vi "Initialize Attributes.vi"(8 "Error In":errorcluster, 10 "Attribute Data":variant, 11 "KIT-QVA in":refnum<class "KIT-QVA.lvclass">) -> (0 "Error Out":errorcluster, 2 "Found?":bool, 3 "KIT-QVA out":refnum<class "KIT-QVA.lvclass">)   [LabVIEW 2014, in "KIT-QVA.lvlib" / "KIT-QVA.lvclass"]
doc: "Initialize object attribute.\n\nUnique resources should be allocated elsewhere!"
uses:
  KIT-QVA.lvclass
  HardwareStatus-PVEnum.ctl
  RackStatus-PVEnum.ctl
  DetectorStatus-PVEnum.ctl
  CSPP_Core/Classes/CS++ProcessVariables/ProcessVariable/PV.lvclass
  CSPP_Core/Classes/CS++ProcessVariables/ProcessVariable/PV.lvclass/PV.ctl
  CSPP_Core/Actors/CS++BaseActor/CS++BaseActor.lvclass/CS++BaseActor.ctl
  KIT-QVA.lvclass/KIT-QVA.ctl
  CSPP_Core/Classes/CS++ProcessVariables/ProcessVariable/Write PV URL.vi
  CSPP_Core/Classes/CS++ProcessVariables/ProcessVariable/Write Type Descriptor.vi
  CSPP_Core/Classes/CS++ProcessVariables/ProcessVariable/Write Name.vi
  CSPP_Core/Actors/CS++DeviceActor/CS++DeviceActor.lvclass
  CSPP_Core/Classes/CS++BaseClasses/Factory/CS++Factory.lvclass
  CSPP_Core/Libraries/Utilities/CS++Utilities.lvlib
  CSPP_Core/Actors/CS++BaseActor/CS++BaseActor.lvclass
  CSPP_Core/Classes/CS++ProcessVariables/CS++ProcessVariables.lvlib
panel:
  in  "Detector-PVEnum":T1
  in  "Rack-PVEnum":T2
  in  "Hardware-PVEnum":T3
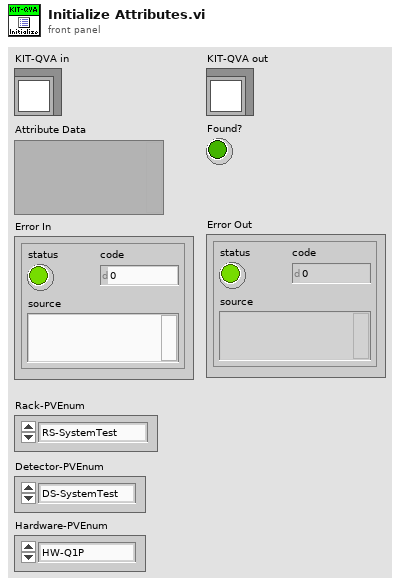
[diagram p1: front panel]
types:
  T1 = typedef "KIT-QVA.lvlib/KIT-QVA.lvclass/DetectorStatus-PVEnum.ctl" = enum16{"DS-SystemTest", "DS-TestMode", "DS-Fault", "DS-Quench", "DS-UTFault", "DS-BusError", "DS-SystemFault", "DS-ADCRaw", "DS-ADCV"}
  T2 = typedef "KIT-QVA.lvlib/KIT-QVA.lvclass/RackStatus-PVEnum.ctl" = enum16{"RS-SystemTest", "RS-TestMode", "RS-Fault", "RS-Quench", "RS-UTFault", "RS-BusError", "RS-SystemFault", "RS-ControlMode", "RS-AveragedT"}
  T3 = typedef "KIT-QVA.lvlib/KIT-QVA.lvclass/HardwareStatus-PVEnum.ctl" = enum16{"HW-Q1P", "HW-Q1M", "HW-Q2P", "HW-Q2M", "HW-Mute", "HW-STestBit", "HW-QD1", "HW-QD2"}
  T4 = cluster{"Q1+":bool, "Q1-":bool, "Q2+":bool, "Q2-":bool, "Mute":bool, "STest-Bit":bool, "QD1":bool, "QD2":bool}
  T5 = cluster{"System Test":bool, "Test Mode":bool, "Fault":bool, "Quench":bool, "U/T Fault":bool, "Bus Error":bool, "System Fault":bool, "Reserved":bool}
  T6 = cluster{"System Test":bool, "Test Mode":bool, "Fault":bool, "Quench":bool, "U/T Fault":bool, "Bus Error":bool, "System Fault":bool, "Control Mode":bool}
  T7 = cluster{"System Test":bool, "Test Mode":bool, "Fault":bool, "Quench":bool, "U/T Fault":bool, "Bus Error":bool, "System Fault":bool, "Reserved":bool}[]
  T8 = cluster{"Q1+":bool, "Q1-":bool, "Q2+":bool, "Q2-":bool, "Mute":bool, "STest-Bit":bool, "QD1":bool, "QD2":bool}[]
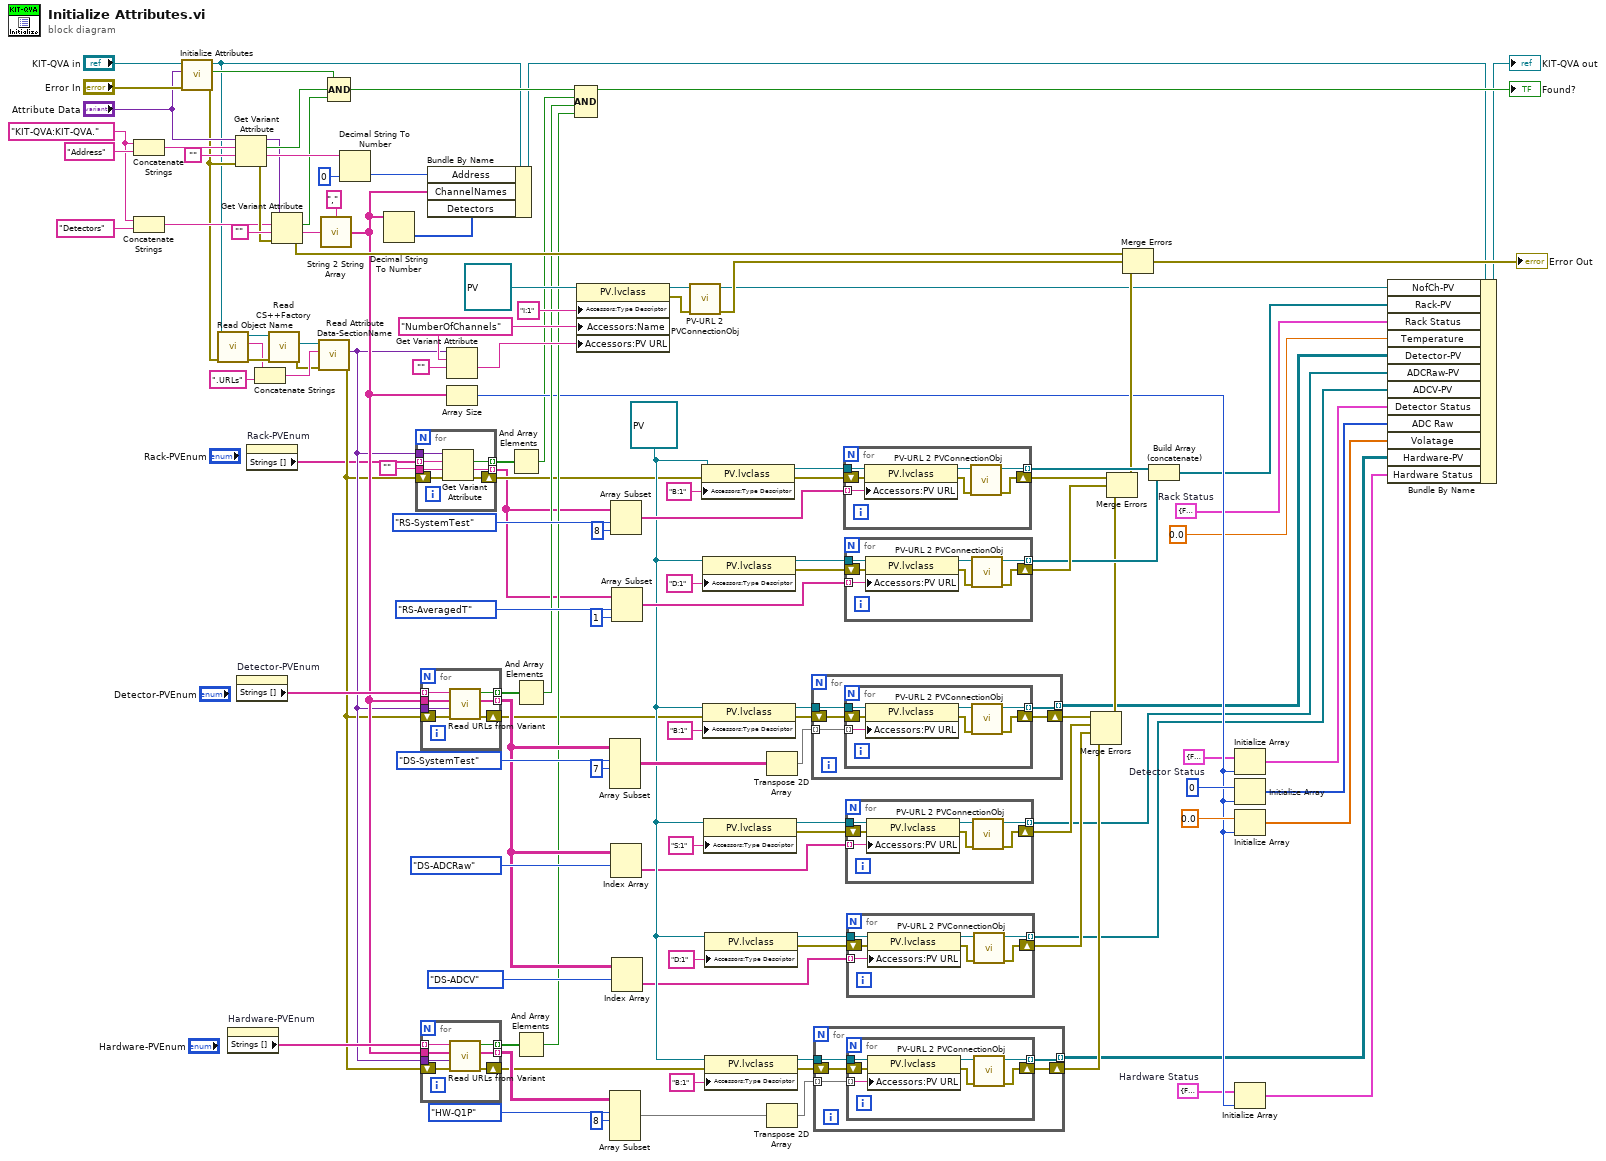
[diagram p0: block diagram]
diagram:
  w16 = T4 {"Q1+"=FALSE, "Q1-"=FALSE, "Q2+"=FALSE, "Q2-"=FALSE, "Mute"=FALSE, "STest-Bit"=FALSE, "QD1"=FALSE, "QD2"=FALSE}  # Hardware Status
  w17 = T5 {"System Test"=FALSE, "Test Mode"=FALSE, "Fault"=FALSE, "Quench"=FALSE, "U/T Fault"=FALSE, "Bus Error"=FALSE, "System Fault"=FALSE, "Reserved"=FALSE}  # Detector Status
  w19 = T6 {"System Test"=FALSE, "Test Mode"=FALSE, "Fault"=FALSE, "Quench"=FALSE, "U/T Fault"=FALSE, "Bus Error"=FALSE, "System Fault"=FALSE, "Control Mode"=FALSE}  # Rack Status
  w41 = refnum<class "PV.lvclass"> refnum ("CS++ProcessVariables.lvlib:PV.lvclass")
  w91 = "NumberOfChannels" ("string")
  w111 = "KIT-QVA:KIT-QVA."
  n1 = Concatenate Strings(w111, "Address" ("string")) -> (w123:string)
  n2 = Concatenate Strings(w111, "Detectors" ("string")) -> (w110:string)
  n3 = call-parent "Initialize Attributes.vi"("error in (no error)"="Error In", "Attribute Data"="Attribute Data", "CS++DeviceActor in"="KIT-QVA in") -> ("error out"=w105:errorcluster, "Found?"=w117:bool, "CS++DeviceActor out"=w104:refnum<class "KIT-QVA.lvclass">)  [unwired: 6 in]
  n4 = call "Read Object Name.vi"("error in (no error)"=w105, "CS++BaseActor in"=w104) -> ("error out"=w103:errorcluster, "Object Name"=w99:string, "CS++BaseActor out"=w106:refnum<class "KIT-QVA.lvclass">)  [unwired: 7 in]
  n5 = property on="Hardware-PVEnum" class="Enum (strict)"() -> ("Strings []"=w40:string[])  [unwired: 2 in, 2 out]
  n6 = Get Variant Attribute(Variant="Attribute Data", name=w123, default value (empty Variant)="", error in=w105) -> (duplicate Variant=w114:variant, found=w118:bool, value=w121:string, error out=w113:errorcluster)
  n7 = property on="Detector-PVEnum" class="Enum (strict)"() -> ("Strings []"=w57:string[])  [unwired: 2 in, 2 out]
  n8 = property on="Rack-PVEnum" class="Enum (strict)"() -> ("Strings []"=w9:string[])  [unwired: 2 in, 2 out]
  n9 = Concatenate Strings(w99, ".URLs" ("string")) -> (w102:string)
  n10 = call "Read CS++Factory.vi"("error in (no error)"=w103, "CS++BaseActor in"=w106) -> ("error out"=w97:errorcluster, "CS++Factory"=w98:refnum<class "CS++Factory.lvclass">)  [unwired: 7 in, 1 out]
  n11 = Get Variant Attribute(Variant=w114, name=w110, default value (empty Variant)="", error in=w113) -> (found=w109:bool, value=w108:string, error out=w73:errorcluster)  [unwired: 1 out]
  n12 = call-dynamic "Read Attribute Data-SectionName.vi"("error in (no error)"=w97, "Object Name"=w102, "CS++Factory in"=w98) -> ("error out"=w11:errorcluster, "Attribute Data"=w12:variant)  [unwired: 6 in, 1 out]
  n13 = call "String 2 String Array.vi"("String"=w108, "Delimiter (\",\")"="," ("Delimiter (\",\")")) -> ("Substrings"=w20:string[])
  n14 = Compound Arithmetic op=AND(w117, w118, w109) -> (w116:bool)
  n15 = Decimal String To Number(string=w121, default (0L)=0 ("default (0 I32)")) -> (number=w120:i32)  [unwired: 1 in, 1 out]
  n16 = Decimal String To Number(string=w20) -> (number=w90:i32[])  [unwired: 2 in, 1 out]
  n17 = for {
    tunnel: [w130] -> w14 mode=indexing
    tunnel: "" -> [w133]
    tunnel: w9 -> [w132] mode=indexing
    shift-right: [w134] -> w15
    shift-left: w11 -> [w131]
    tunnel: [w128] -> w13 mode=indexing
    tunnel: w12 -> [w129]
    n18 = Get Variant Attribute(Variant=w129, name=w132, default value (empty Variant)=w133, error in=w131) -> (found=w130:bool, value=w128:string, error out=w134:errorcluster)  [unwired: 1 out]
  }
  n19 = for {
    tunnel: w57 -> [w141] mode=indexing
    tunnel: [w140] -> w59 mode=indexing
    tunnel: w12 -> [w138]
    tunnel: w20 -> [w137]
    tunnel: [w136] -> w50 mode=indexing
    shift-right: [w139] -> w22
    shift-left: w11 -> [w135]
    n20 = call "Read URLs from Variant.vi"("Error In"=w135, "URL Section Data"=w138, "Channel Names"=w137, "URL Prefix"=w141) -> ("Error Out"=w139:errorcluster, "URLs"=w136:string[], "Found?"=w140:bool)  [unwired: 5 in]
  }
  n21 = for {
    tunnel: w40 -> [w148] mode=indexing
    tunnel: [w147] -> w48 mode=indexing
    tunnel: w12 -> [w145]
    tunnel: w20 -> [w144]
    tunnel: [w143] -> w42 mode=indexing
    shift-right: [w146] -> w21
    shift-left: w11 -> [w142]
    n22 = call "Read URLs from Variant.vi"("Error In"=w142, "URL Section Data"=w145, "Channel Names"=w144, "URL Prefix"=w148) -> ("Error Out"=w146:errorcluster, "URLs"=w143:string[], "Found?"=w147:bool)  [unwired: 5 in]
  }
  n23 = Bundle By Name(cluster=w104, "Address"=w120, "ChannelNames"=w20, "Detectors"=w90) -> (w34:refnum<class "KIT-QVA.lvclass">)
  n24 = Get Variant Attribute(Variant=w12, name=w91, default value (empty Variant)="") -> (value=w92:string)  [unwired: 1 in, 3 out]
  n25 = Array Size(array=w20) -> (size(s)=w26:i32)
  n26 = And Array Elements(Boolean array=w14) -> (logical AND=w8:bool)
  n27 = And Array Elements(Boolean array=w59) -> (logical AND=w36:bool)
  n28 = And Array Elements(Boolean array=w48) -> (logical AND=w35:bool)
  n29 = Compound Arithmetic op=AND(w116, w8, w36, w35) -> (→"Found?":bool)
  n30 = property class="PV.lvclass"(reference=refnum<class "PV.lvclass"> refnum ("CS++ProcessVariables.lvlib:PV.lvclass"), "Accessors:Type Descriptor"="I:1" ("Type Descriptor"), "Accessors:Name"=w91, "Accessors:PV URL"=w92) -> (reference out=w96:refnum<class "PV.lvclass">, error out=w95:errorcluster)  [unwired: 1 in]
  n31 = Array Subset(array=w50, index (row)=DetectorStatus-PVEnum."DS-SystemTest" ("Detector-PVEnum"), length (row)=7 ("length")) -> (w64:string[][])  [unwired: 2 in]
  n32 = Array Subset(array=w42, index (row)=HardwareStatus-PVEnum."HW-Q1P" ("Hardware-PVEnum"), length (row)=8 ("length")) -> (w44:string[][])  [unwired: 2 in]
  n33 = Array Subset(array=w13, index=RackStatus-PVEnum."RS-SystemTest" ("Rack-PVEnum"), length=8) -> (w84:string[])
  n34 = Index Array(array=w50, index (row)=DetectorStatus-PVEnum."DS-ADCRaw" ("Detector-PVEnum")) -> (element=w5:string[])  [unwired: 1 in]
  n35 = Array Subset(array=w13, index=RackStatus-PVEnum."RS-AveragedT" ("Rack-PVEnum"), length=1) -> (w81:string[])
  n36 = Index Array(array=w50, index (row)=DetectorStatus-PVEnum."DS-ADCV" ("Detector-PVEnum")) -> (element=w4:string[])  [unwired: 1 in]
  n37 = call "PV-URL 2 PVConnectionObj.vi"("Error In"=w95, "PV"=w96) -> ("Error Out"=w71:errorcluster, "PVConnection"=w32:refnum<class "PVConnection.lvclass">)  [unwired: 7 in, 1 out]
  n38 = property class="PV.lvclass"(reference=w41, error in=w15, "Accessors:Type Descriptor"="B:1" ("Type Descriptor")) -> (reference out=w86:refnum<class "PV.lvclass">, error out=w87:errorcluster)
  n39 = property class="PV.lvclass"(reference=w41, "Accessors:Type Descriptor"="D:1" ("Type Descriptor")) -> (reference out=w79:refnum<class "PV.lvclass">, error out=w78:errorcluster)  [unwired: 1 in]
  n40 = property class="PV.lvclass"(reference=w41, error in=w22, "Accessors:Type Descriptor"="B:1" ("Type Descriptor")) -> (reference out=w62:refnum<class "PV.lvclass">, error out=w61:errorcluster)
  n41 = property class="PV.lvclass"(reference=w41, "Accessors:Type Descriptor"="S:1" ("Type Descriptor")) -> (reference out=w67:refnum<class "PV.lvclass">, error out=w68:errorcluster)  [unwired: 1 in]
  n42 = property class="PV.lvclass"(reference=w41, "Accessors:Type Descriptor"="D:1" ("Type Descriptor")) -> (reference out=w52:refnum<class "PV.lvclass">, error out=w51:errorcluster)  [unwired: 1 in]
  n43 = property class="PV.lvclass"(reference=w41, error in=w21, "Accessors:Type Descriptor"="B:1" ("Type Descriptor")) -> (reference out=w46:refnum<class "PV.lvclass">, error out=w47:errorcluster)
  n44 = Transpose 2D Array(2D array=w64) -> (transposed array=w7:string[][])
  n45 = Transpose 2D Array(2D array=w44) -> (transposed array=w6:string[][])
  n46 = for {
    tunnel: w62 -> [w153]
    tunnel: w7 -> [w152] mode=indexing
    tunnel: [w151] -> w3 mode=indexing
    shift-right: [w150] -> w60
    shift-left: w61 -> [w149]
    n47 = for {
      tunnel: w153 -> [w159]
      tunnel: w152 -> [w158] mode=indexing
      tunnel: [w157] -> w151 mode=indexing
      shift-right: [w156] -> w150
      shift-left: w149 -> [w154]
      n48 = property class="PV.lvclass"(reference=w159, error in=w154, "Accessors:PV URL"=w158) -> (reference out=w160:refnum<class "PV.lvclass">, error out=w155:errorcluster)
      n49 = call "PV-URL 2 PVConnectionObj.vi"("Error In"=w155, "PV"=w160) -> ("Error Out"=w156:errorcluster, "PVConnection"=w157:refnum<class "PVConnection.lvclass">)  [unwired: 7 in, 1 out]
    }
  }
  n50 = for {
    tunnel: w46 -> [w165]
    tunnel: w6 -> [w164] mode=indexing
    tunnel: [w163] -> w23 mode=indexing
    shift-right: [w162] -> w38
    shift-left: w47 -> [w161]
    n51 = for {
      tunnel: w165 -> [w171]
      tunnel: w164 -> [w170] mode=indexing
      tunnel: [w169] -> w163 mode=indexing
      shift-right: [w168] -> w162
      shift-left: w161 -> [w166]
      n52 = property class="PV.lvclass"(reference=w171, error in=w166, "Accessors:PV URL"=w170) -> (reference out=w172:refnum<class "PV.lvclass">, error out=w167:errorcluster)
      n53 = call "PV-URL 2 PVConnectionObj.vi"("Error In"=w167, "PV"=w172) -> ("Error Out"=w168:errorcluster, "PVConnection"=w169:refnum<class "PVConnection.lvclass">)  [unwired: 7 in, 1 out]
    }
  }
  n54 = for {
    tunnel: w86 -> [w178]
    tunnel: w84 -> [w177] mode=indexing
    tunnel: [w176] -> w89 mode=indexing
    shift-right: [w175] -> w88
    shift-left: w87 -> [w173]
    n55 = property class="PV.lvclass"(reference=w178, error in=w173, "Accessors:PV URL"=w177) -> (reference out=w179:refnum<class "PV.lvclass">, error out=w174:errorcluster)
    n56 = call "PV-URL 2 PVConnectionObj.vi"("Error In"=w174, "PV"=w179) -> ("Error Out"=w175:errorcluster, "PVConnection"=w176:refnum<class "PVConnection.lvclass">)  [unwired: 7 in, 1 out]
  }
  n57 = for {
    tunnel: w79 -> [w185]
    tunnel: w81 -> [w184] mode=indexing
    tunnel: [w183] -> w74 mode=indexing
    shift-right: [w182] -> w75
    shift-left: w78 -> [w180]
    n58 = property class="PV.lvclass"(reference=w185, error in=w180, "Accessors:PV URL"=w184) -> (reference out=w186:refnum<class "PV.lvclass">, error out=w181:errorcluster)
    n59 = call "PV-URL 2 PVConnectionObj.vi"("Error In"=w181, "PV"=w186) -> ("Error Out"=w182:errorcluster, "PVConnection"=w183:refnum<class "PVConnection.lvclass">)  [unwired: 7 in, 1 out]
  }
  n60 = for {
    tunnel: w67 -> [w192]
    tunnel: w5 -> [w191] mode=indexing
    tunnel: [w190] -> w2 mode=indexing
    shift-right: [w189] -> w69
    shift-left: w68 -> [w187]
    n61 = property class="PV.lvclass"(reference=w192, error in=w187, "Accessors:PV URL"=w191) -> (reference out=w193:refnum<class "PV.lvclass">, error out=w188:errorcluster)
    n62 = call "PV-URL 2 PVConnectionObj.vi"("Error In"=w188, "PV"=w193) -> ("Error Out"=w189:errorcluster, "PVConnection"=w190:refnum<class "PVConnection.lvclass">)  [unwired: 7 in, 1 out]
  }
  n63 = for {
    tunnel: w52 -> [w199]
    tunnel: w4 -> [w198] mode=indexing
    tunnel: [w197] -> w1 mode=indexing
    shift-right: [w196] -> w49
    shift-left: w51 -> [w194]
    n64 = property class="PV.lvclass"(reference=w199, error in=w194, "Accessors:PV URL"=w198) -> (reference out=w200:refnum<class "PV.lvclass">, error out=w195:errorcluster)
    n65 = call "PV-URL 2 PVConnectionObj.vi"("Error In"=w195, "PV"=w200) -> ("Error Out"=w196:errorcluster, "PVConnection"=w197:refnum<class "PVConnection.lvclass">)  [unwired: 7 in, 1 out]
  }
  n66 = Merge Errors(w60, w69, w49, w38) -> (w58:errorcluster)
  n67 = Merge Errors(w88, w75, w58) -> (w70:errorcluster)
  n68 = Merge Errors(w73, w71, w70) -> (→"Error Out":errorcluster)
  n69 = Build Array (concatenate)(w89, w74) -> (w24:refnum<class "PVConnection.lvclass">[])
  n70 = Initialize Array(w17, w26) -> (w29:T7)
  n71 = Initialize Array(i16 0 ("ADC Raw"), w26) -> (w28:i16[])
  n72 = Initialize Array(dbl[unit] 0.0 ("Volatage"), w26) -> (w27:dbl[unit][])
  n73 = Initialize Array(w16, w26) -> (w25:T8)
  n74 = Bundle By Name(cluster=w34, "NofCh-PV"=w32, "Rack-PV"=w24, "Rack Status"=w19, "Temperature"=dbl[unit] 0.0, "Detector-PV"=w3, "ADCRaw-PV"=w2, "ADCV-PV"=w1, "Detector Status"=w29, "ADC Raw"=w28, "Volatage"=w27, "Hardware-PV"=w23, "Hardware Status"=w25) -> (→"KIT-QVA out":refnum<class "KIT-QVA.lvclass">)
